vi "Gyro Begin.vi"() -> ()   [LabVIEW 2011]
uses:
  <vilib>/Rock Robotics/SystemInterfaces/AI/FPGA_AIGyroChannel.ctl
  Robot Global Data.vi
panel:
  in  "Steering Gain (VoltsPerDegree/Second)":dbl=0.0125
  in  "Gain (VoltsPerDegree/Second)":dbl=0.0125
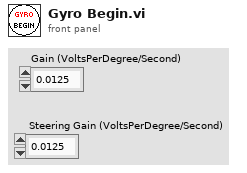
[diagram p1: front panel]
types:
  T1 = typedef "FPGA_AIGyroChannel.ctl" = enum8{"AI 1", "AI 2", "Invalid"}
  T2 = typedef "WPI_GyroDevRef.ctl" = cluster{"DevStatus":errorcluster, "Analog Module":T3, "Analog Channel":T4, "Offset":dbl, "Gain (VoltsPerDegree/Second)":dbl}
  T3 = typedef "FPGA_TypedefAnalogModule.ctl" = enum16{"Analog Module 1", "Analog Module 2"}
  T4 = typedef "FPGA_AIChannel.ctl" = enum8{"AI 1", "AI 2", "AI 3", "AI 4", "AI 5", "AI 6", "AI 7", "AI 8", "Invalid"}
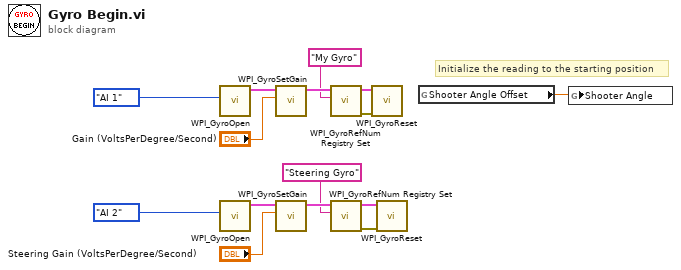
[diagram p0: block diagram]
diagram:
  # "Initialize the reading to the starting position"
  n1 = call <vilib>:"WPI_GyroOpen.vi"("Analog Channel"=FPGA_AIGyroChannel."AI 1") -> ("GyroDevRef"=w14:T2)  [unwired: 8 in, 2 out]
  n2 = call <vilib>:"WPI_GyroOpen.vi"("Analog Channel"=FPGA_AIGyroChannel."AI 2") -> ("GyroDevRef"=w9:T2)  [unwired: 8 in, 2 out]
  n3 = call <vilib>:"WPI_GyroSetGain.vi"("Gain (VoltsPerDegree/Second)"="Gain (VoltsPerDegree/Second)", "GyroDevRef"=w14) -> ("GyroDevRef"=w12:T2)  [unwired: 8 in, 1 out]
  n4 = call <vilib>:"WPI_GyroSetGain.vi"("Gain (VoltsPerDegree/Second)"="Steering Gain (VoltsPerDegree/Second)", "GyroDevRef"=w9) -> ("GyroDevRef"=w7:T2)  [unwired: 8 in, 1 out]
  n5 = call <vilib>:"WPI_GyroRefNum Registry Set.vi"("refnum name"="My Gyro", "GyroDevRef"=w12) -> ("error out"=w5:errorcluster, "GyroDevRef"=w4:T2)  [unwired: 8 in]
  n6 = call <vilib>:"WPI_GyroRefNum Registry Set.vi"("refnum name"="Steering Gyro", "GyroDevRef"=w7) -> ("error out"=w2:errorcluster, "GyroDevRef"=w3:T2)  [unwired: 8 in]
  n7 = call <vilib>:"WPI_GyroReset.vi"("error in (no error)"=w5, "GyroDevRef"=w4) -> ()  [unwired: 8 in, 2 out]
  n8 = call <vilib>:"WPI_GyroReset.vi"("error in (no error)"=w2, "GyroDevRef"=w3) -> ()  [unwired: 8 in, 2 out]
  n9 = global read "Robot Global Data.vi" "Shooter Angle Offset"() -> (w1:dbl)
  n10 = global write "Robot Global Data.vi" "Shooter Angle"(w1) -> ()
